vi "dfd_FXP PtByPt Lattice MA.vi"(6 "state in":i64[](array[numeric]), 7 "FXPOPs":T6[](array[typedef]) {"source" items=["Coef a/k"=0, "Coef b/v"=7, "Input"=1, "Output"=2, "Multiplicand"=3, "Product"=4, "Sum"=5, "Delay"=6, "Gain"=8]}, 8 "filtering statistics in":T4(array[cluster]) {"statistics information"."min value" format="%.2f"; "statistics information"."max value" format="%.2f"; "Quantizer Source" items=["Coefficients a/k"=0, "Coefficients b/v"=7, "Input"=1, "Output"=2, "Multiplicand"=3, "Product"=4, "Sum"=5, "Delay"=6]}, 10 "coef k[M..1]":T5, 11 "x":T1={"value"=0, "wl"=0, "iwl"=0, "Signed"=TRUE} {"value" format="%.0x"}) -> (0 "filtering statistics out":T4(array[cluster]) {"statistics information"."min value" format="%.2f"; "statistics information"."max value" format="%.2f"; "Quantizer Source" items=["Coefficients a/k"=0, "Coefficients b/v"=7, "Input"=1, "Output"=2, "Multiplicand"=3, "Product"=4, "Sum"=5, "Delay"=6]}, 2 "max phase filtered x":T1={"value"=0, "wl"=0, "iwl"=0, "Signed"=TRUE} {"value" format="%.0x"}, 3 "min phase filtered x":T1={"value"=0, "wl"=0, "iwl"=0, "Signed"=TRUE} {"value" format="%.0x"}, 4 "state out":i64[](array[numeric]))   [LabVIEW 2017, in "NI_DigFilter_FXP.lvlib"]
uses:
  <vilib>/addons/Digital Filter Design/NI_DigFilter_FXP.lvlib
  <vilib>/addons/Digital Filter Design/_Objects.llb/dfd_DFXP Data Type (scaler).ctl
  <vilib>/addons/Digital Filter Design/_Objects.llb/dfd_DFXP Operation Parameter.ctl
  <vilib>/addons/Digital Filter Design/_Objects.llb/dfd_Internal Quantization Srcs.ctl
  <vilib>/addons/Digital Filter Design/_Objects.llb/dfd_DFXP Data Type (vector).ctl
  <vilib>/addons/Digital Filter Design/_Objects.llb/DFD Quantization Sources.ctl
  <vilib>/addons/Digital Filter Design/_Objects.llb/DFD FXP Statistics Data.ctl
  <vilib>/addons/Digital Filter Design/NI_DigFilterLicensed.lvlib
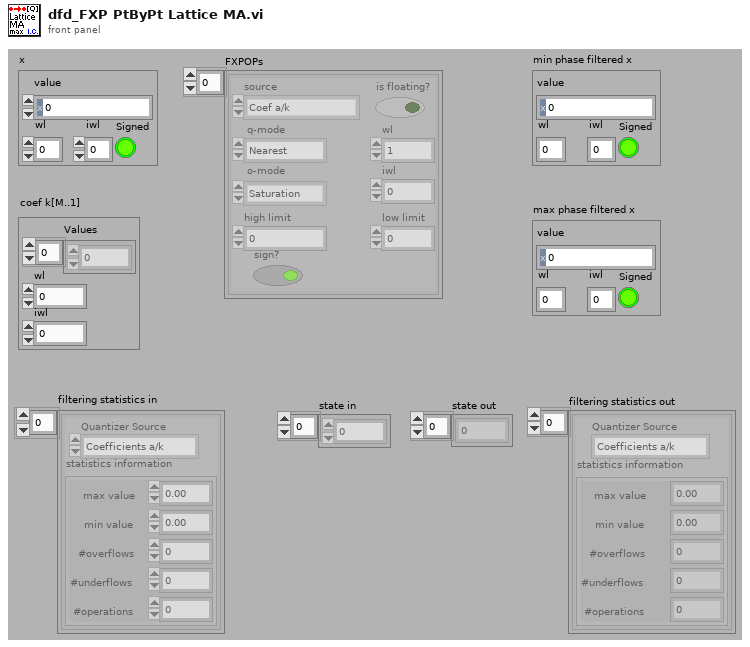
[diagram p1: front panel]
types:
  T1 = typedef "dfd_DFXP Data Type (scaler).ctl" = cluster{"value":i64, "wl":i16, "iwl":i16, "Signed":bool}
  T2 = typedef "NI_DigFilterLicensed.lvlib/DFD Quantization Sources.ctl" = u16
  T3 = typedef "NI_DigFilterLicensed.lvlib/DFD FXP Statistics Data.ctl" = cluster{"max value":ext, "min value":ext, "#overflows":i32, "#underflows":i32, "#operations":i32}
  T4 = cluster{"Quantizer Source":T2, "statistics information":T3}[]
  T5 = typedef "dfd_DFXP Data Type (vector).ctl" = cluster{"Values":i64[], "wl":i16, "iwl":i16}
  T6 = typedef "dfd_DFXP Operation Parameter.ctl" = cluster{"source":T7, "is floating?":bool, "o-mode":enum16{"Saturation", "Wrap"}, "q-mode":enum16{"Nearest", "Truncation"}, "wl":i16, "high limit":i64, "low limit":i64, "iwl":i16, "sign?":bool}
  T7 = typedef "NI_DigFilterLicensed.lvlib/dfd_Internal Quantization Srcs.ctl" = u16
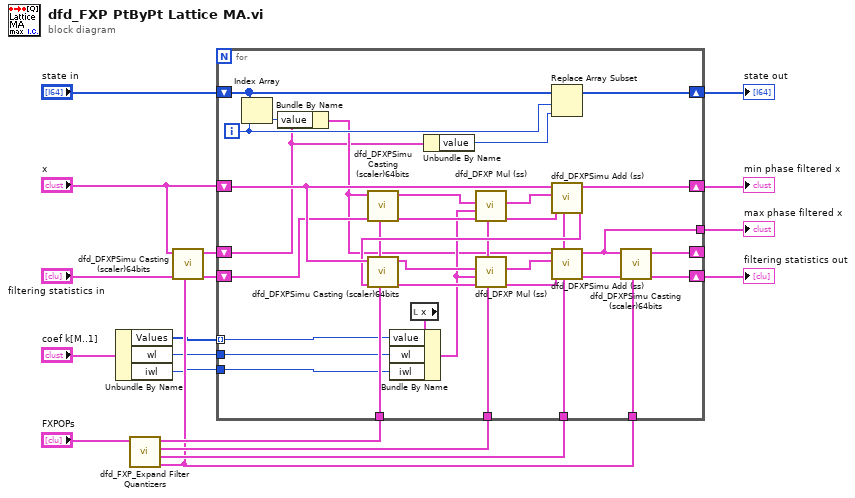
[diagram p0: block diagram]
diagram:
  n1 = Unbundle By Name("coef k[M..1]") -> ("Values"=w3:i64[], "wl"=w2:i16, "iwl"=w1:i16)
  n2 = call <vilib>:"dfd_FXP_Expand Filter Quantizers.vi"("FXPOPs"="FXPOPs") -> ("Delay"=w7:T6, "Sum"=w12:T6, "Product"=w13:T6, "Multiplicand"=w14:T6)  [unwired: 7 out]
  n3 = call <vilib>:"dfd_DFXPSimu Casting (scaler)64bits.vi"("op params"=w7, "filtering statistics in"="filtering statistics in", "Value in"="x") -> ("filtering statistics out"=w9:T4, "Value out"=w18:T1)  [unwired: 1 in, 6 out]
  n4 = for {
    shift-right: [w46] -> w6
    shift-left: "x" -> [w42]
    shift-right: [w45] -> _
    shift-left: w18 -> [w19]
    shift-right: [w50] -> w16
    shift-left: "state in" -> [w49]
    tunnel: [w41] -> w15
    tunnel: w14 -> [w31]
    tunnel: w13 -> [w29]
    tunnel: w12 -> [w30]
    tunnel: w7 -> [w32]
    shift-right: [w33] -> w8
    shift-left: w9 -> [w40]
    tunnel: w3 -> [w26] mode=indexing
    tunnel: w2 -> [w23]
    tunnel: w1 -> [w22]
    i -> [w48]
    n5 = Index Array(array=w49, index=w48) -> (element=w43:i64)
    n6 = Bundle By Name(cluster=w19, "value"=w43) -> (w20:T1)
    n7 = call <vilib>:"dfd_DFXPSimu Casting (scaler)64bits.vi"("op params"=w31, "filtering statistics in"=w40, "Value in"=w20) -> ("filtering statistics out"=w39:T4, "Value out"=w28:T1)  [unwired: 1 in, 6 out]
    n8 = local read "x"() -> (w24:T1)
    n9 = Bundle By Name(cluster=w24, "value"=w26, "wl"=w23, "iwl"=w22) -> (w25:T1)
    n10 = Unbundle By Name(w19) -> ("value"=w21:i64)
    n11 = call <vilib>:"dfd_DFXP Mul (ss).vi"("op params"=w29, "filtering statistics in"=w39, "Value in 2"=w25, "Value in"=w28) -> ("filtering statistics out"=w38:T4, "Value out"=w47:T1)  [unwired: 6 out]
    n12 = Replace Array Subset(array=w49, new element=w21, index=w48) -> (w50:i64[])
    n13 = call <vilib>:"dfd_DFXPSimu Add (ss).vi"("op params"=w30, "filtering statistics in"=w38, "value in 2"=w47, "value in 1"=w42) -> ("filtering statistics out"=w37:T4, "value out"=w46:T1)  [unwired: 1 in, 5 out]
    n14 = call <vilib>:"dfd_DFXPSimu Casting (scaler)64bits.vi"("op params"=w31, "filtering statistics in"=w37, "Value in"=w42) -> ("filtering statistics out"=w36:T4, "Value out"=w27:T1)  [unwired: 2 in, 5 out]
    n15 = call <vilib>:"dfd_DFXP Mul (ss).vi"("op params"=w29, "filtering statistics in"=w36, "Value in 2"=w25, "Value in"=w27) -> ("filtering statistics out"=w35:T4, "Value out"=w44:T1)  [unwired: 6 out]
    n16 = call <vilib>:"dfd_DFXPSimu Add (ss).vi"("op params"=w30, "filtering statistics in"=w35, "value in 2"=w44, "value in 1"=w20) -> ("filtering statistics out"=w34:T4, "value out"=w41:T1)  [unwired: 1 in, 5 out]
    n17 = call <vilib>:"dfd_DFXPSimu Casting (scaler)64bits.vi"("op params"=w32, "filtering statistics in"=w34, "Value in"=w41) -> ("filtering statistics out"=w33:T4, "Value out"=w45:T1)  [unwired: 2 in, 5 out]
  }
  "state out" <- w16
  "max phase filtered x" <- w15
  "filtering statistics out" <- w8
  "min phase filtered x" <- w6
